vi "Simulations Config.vi"(8 "error in (no error)":errorcluster, 11 "FileConfig in":refnum<class "FileConfig.lvclass">) -> (0 "error out":errorcluster, 1 "Found?":bool, 2 "Simulated Classes":T1, 3 "FileConfig out":refnum<class "FileConfig.lvclass">)   [LabVIEW 2019, in "Config.lvlib" / "FileConfig.lvclass"]
doc: "This method reads the simulation constants for the file. The default values are all not simulated.\nThis method does not fail with error if a system is not found. Rather, it just sets it as not/simulated (FALSE)"
uses:
  FileConfig.lvclass
  Config/Controls/Simulated Classes.ctl
  Config.lvclass
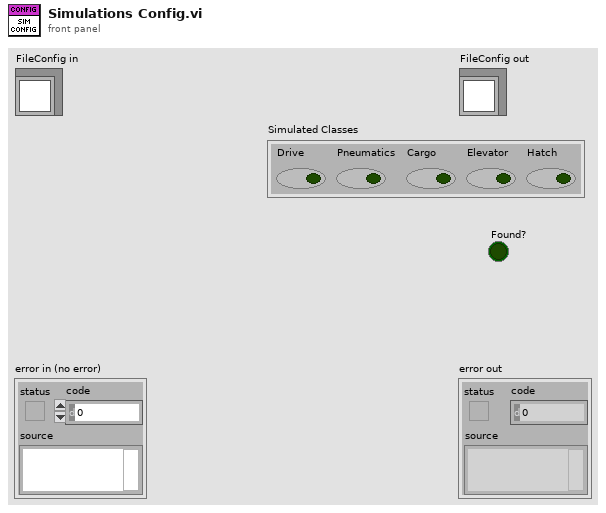
[diagram p1: front panel]
types:
  T1 = typedef "Config.lvlib/Config.lvclass/Simulated Classes.ctl" = cluster{"Drive":bool, "Pneumatics":bool, "Cargo":bool, "Elevator":bool, "Hatch":bool}
  T2 = cluster{"Found Booleans[0]":bool, "Found Booleans[1]":bool, "Found Booleans[2]":bool, "Found Booleans[3]":bool, "Found Booleans[4]":bool}
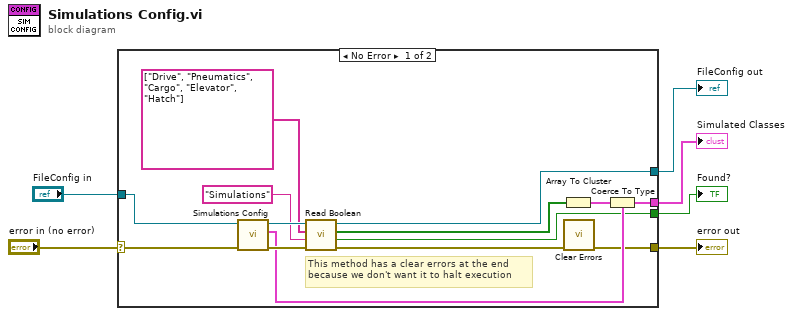
[diagram p0: block diagram]
diagram:
  n1 = case shown="No Error" "error in (no error)" {
    selector: "error in (no error)" -> [w20 w21]
    tunnel: "FileConfig in" -> [w19 w22]
    tunnel: [w7 w21] -> w4
    tunnel: [w15 w22] -> w3
    tunnel: [w9 _] -> w2
    tunnel: [w8 _] -> w1
    frame No Error {
      # "This method has a clear errors at the end\nbecause we don't want it to halt execution"
      n2 = call-parent "Simulations Config.vi"("error in (no error)"=w20, "Config in"=w19) -> ("error out"=w18:errorcluster, "Simulated Classes"=w10:T1, "Config out"=w16:refnum<class "FileConfig.lvclass">)  [unwired: 6 in, 1 out]
      n3 = call "Read Boolean.vi"("error in (no error)"=w18, "section"="Simulations", "keys"=string[] ["Drive", "Pneumatics", "Cargo", "Elevator", "Hatch"], "FileConfig in"=w16) -> ("error out"=w17:errorcluster, "Found?"=w8:bool, "Found Booleans"=w12:bool[], "FileConfig out"=w15:refnum<class "FileConfig.lvclass">)  [unwired: 4 in]
      n4 = Array To Cluster(array=w12) -> (cluster=w11:T2)
      n5 = call <vilib>:"Clear Errors.vi"("error in (no error)"=w17) -> ("error out"=w7:errorcluster)  [unwired: 5 in, 1 out]
      n6 = Coerce To Type(0:w11, 1:w10) -> (2:w9:T1)
    }
    frame Error {
    }
  }
  "error out" <- w4
  "FileConfig out" <- w3
  "Simulated Classes" <- w2
  "Found?" <- w1
